vi "Place Noeds and Engine Global.vi"() -> ()   [LabVIEW 2014, in "Initialization and IO Node Scripting.lvlib"]
uses:
  Initialization and IO Node Scripting.lvlib
panel:
  in  "Place Nodes and Engine":bool
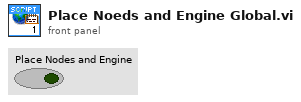
[diagram p1: front panel]
diagram:
